vi "GOMDBTS2048 calib Az Get Calib Lamp.vi"(8 "error in (no error)":errorcluster, 11 "handle":i32) -> (0 "error out":errorcluster, 1 "function return":i32, 2 "name":string, 3 "values":dbl[](array[numeric]))   [LabVIEW 2015, in "GOMDBTS2048.lvlib"]
doc: "GOBTS2048DLL int __stdcall GOMDBTS2048_calibTristimulusSetXYZ(int handle, double* valuesX, double* valuesY, double* valuesZ); GOBTS2048DLL int __stdcall GOMDBTS2048_calibTristimulusGetXYZ(int handle, double* valuesX, double* valuesY, double* valuesZ); GOBTS2048DLL int __stdcall GOMDBTS2048_calibAzSetCalibLamp(int handle, double* values, char* name); GOBTS2048DLL int __stdcall GOMDBTS2048_calibAzGetCalibLamp(int handle, double* values, char* name);"
uses:
  GOMDBTS2048.lvlib
  runtime/GOMDBTS2048.dll
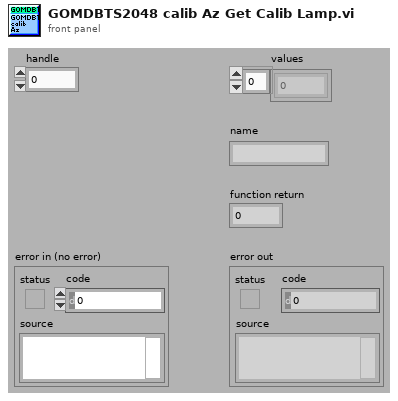
[diagram p1: front panel]
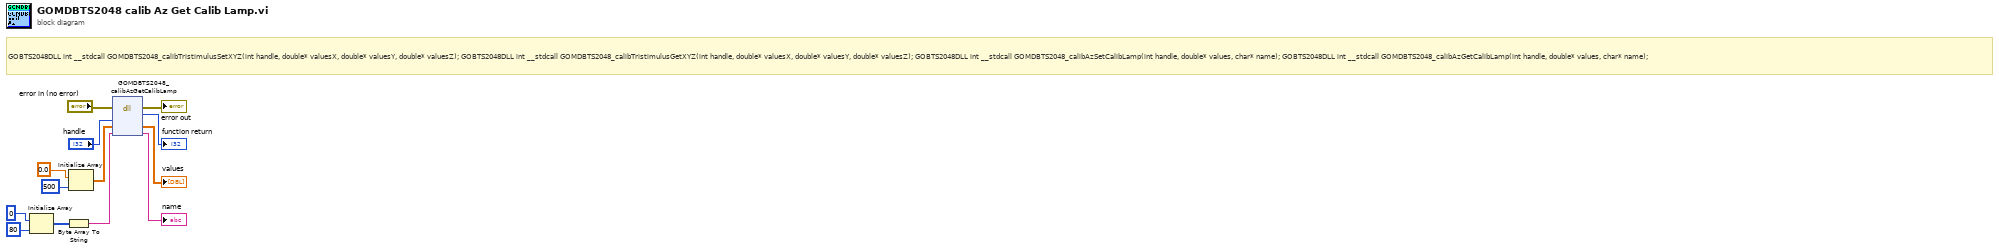
[diagram p0: block diagram]
diagram:
  # "GOBTS2048DLL int __stdcall GOMDBTS2048_calibTristimulusSetXYZ(int handle, double* valuesX, double* valuesY, double* valuesZ); GOBTS2048DLL int __stdcall GOMDBTS2048_calibTristimulusGetXYZ(int handle, double* valuesX, double* valuesY, double* valuesZ); GOBTS2048DLL int __stdcall GOMDBTS2048_calibAzSetCalibLamp(int handle, double* values, char* name); GOBTS2048DLL int __stdcall GOMDBTS2048_calibAzGetCalibLamp(int handle, double* values, char* name);"
  n1 = Initialize Array(u8 0 ("element"), 80 ("dimension size")) -> (w7:u8[])
  n2 = Byte Array To String(unsigned byte array=w7) -> (string=w6:string)
  n3 = Initialize Array(0.0 ("element"), 500 ("dimension size")) -> (w11:dbl[])
  n4 = dll-call lib="C:/Users/rkoch/Documents/GO_Library/runtime/GOMDBTS2048.*" fn="GOMDBTS2048_calibAzGetCalibLamp"(error in="error in (no error)", "handle"="handle", "values"=w11, "name"=w6) -> (error out=→"error out":errorcluster, →"function return":i32, "values"=→"values":dbl[], "name"=→"name":string)  [unwired: 3 in, 1 out]
